vi "Configure Recorder Output.vi.vi"(5 "CALC Block (F: Disable)":bool, 6 "Enable Recorder Output (F: Disable)":bool, 7 "Maximum Power (20 dBm or Watt or %)":dbl=20.0, 8 "error in (no error)":errorcluster, 9 "Minimum Power (-150 dBm or Watt or %)":dbl=-150.0, 10 "Enable Recorder Autoscaling (F: Disable)":bool, 11 "VISA resource name":refnum<visa-resource-name>) -> (0 "error out":errorcluster, 3 "VISA resource name out":refnum<visa-resource-name>)   [LabVIEW 2011, in "Agilent N432A.lvlib"]
doc: "Enables/disables the recorder output and sets the minimum scaling value and maximum scaling value for the specified recorder output."
uses:
  <instrlib>/Agilent N432A/Agilent N432A.lvlib
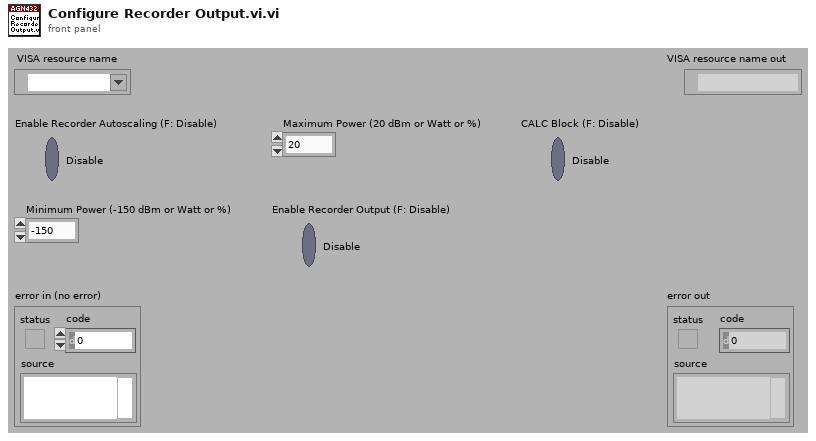
[diagram p1: front panel]
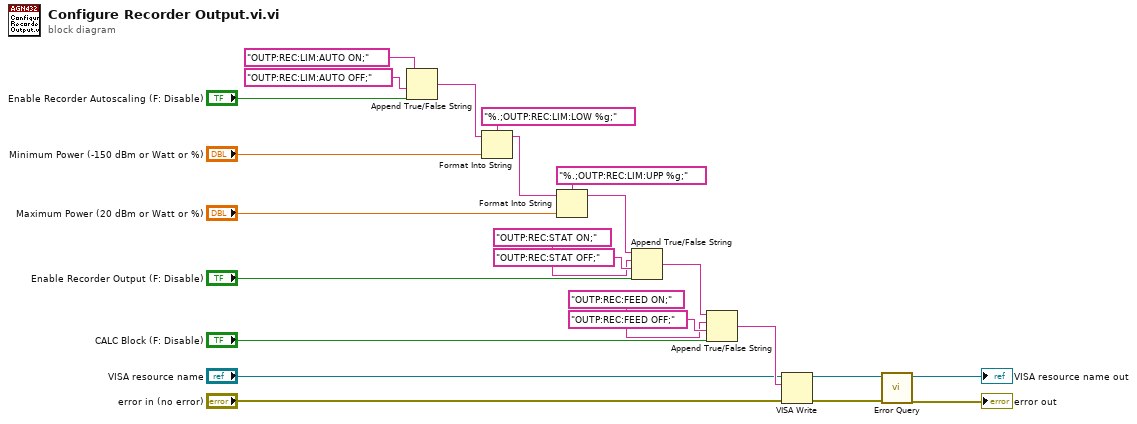
[diagram p0: block diagram]
diagram:
  n1 = Append True/False String(1:"Enable Recorder Autoscaling (F: Disable)", 2:"OUTP:REC:LIM:AUTO OFF;", 3:"OUTP:REC:LIM:AUTO ON;") -> (0:w21:string)  [unwired: 1 in]
  n2 = Format Into String(format string="%.;OUTP:REC:LIM:LOW %g;", initial string=w21, "Minimum Power (-150 dBm or Watt or %)") -> (resulting string=w18:string)  [unwired: 1 in, 1 out]
  n3 = Format Into String(format string="%.;OUTP:REC:LIM:UPP %g;", initial string=w18, "Maximum Power (20 dBm or Watt or %)") -> (resulting string=w15:string)  [unwired: 1 in, 1 out]
  n4 = Append True/False String(1:"Enable Recorder Output (F: Disable)", 2:"OUTP:REC:STAT OFF;", 3:"OUTP:REC:STAT ON;", 4:w15) -> (0:w11:string)
  n5 = Append True/False String(1:"CALC Block (F: Disable)", 2:"OUTP:REC:FEED OFF;", 3:"OUTP:REC:FEED ON;", 4:w11) -> (0:w7:string)
  n6 = VISA Write(VISA resource name="VISA resource name", write buffer=w7, error in (no error)="error in (no error)") -> (VISA resource name out=w4:refnum<visa-resource-name>, error out=w3:errorcluster)  [unwired: 1 out]
  n7 = call <instrlib>:"Error Query.vi"("error in (no error)"=w3, "VISA resource name"=w4) -> ("error out"=→"error out":errorcluster, "VISA resource name out"=→"VISA resource name out":refnum<visa-resource-name>)  [unwired: 6 in, 2 out]
